vi "Is Control Present.vi"(8 "Error In":errorcluster, 10 "Control label":string, 11 "VI ref":refnum<vi>) -> (0 "Error Out":errorcluster, 2 "Present":bool, 3 "VI ref out":refnum<vi>)   [LabVIEW 2015]
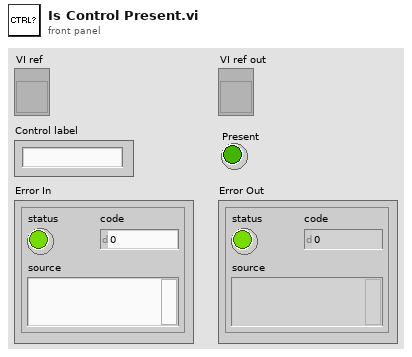
[diagram p1: front panel]
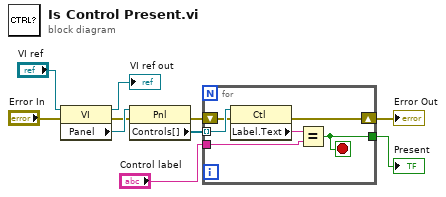
[diagram p0: block diagram]
diagram:
  n1 = property class="VI"(reference="VI ref", error in="Error In") -> (reference out=→"VI ref out":refnum<vi>, error out=w6:errorcluster, "Panel"=w9:refnum<vi>)
  n2 = property class="Pnl"(reference=w9, error in=w6) -> (error out=w5:errorcluster, "Controls[]"=w8:refnum<vi>[])  [unwired: 1 out]
  n3 = for {
    tunnel: w8 -> [w16] mode=indexing
    shift-right: [w14] -> w3
    shift-left: w5 -> [w15]
    tunnel: "Control label" -> [w12]
    tunnel: [w11] -> w2
    stop <- w11 stop-if-true
    n4 = property class="Ctl"(reference=w16, error in=w15) -> (error out=w14:errorcluster, "Label.Text"=w13:string)  [unwired: 1 out]
    n5 = Equal?(x=w13, y=w12) -> (x = y?=w11:bool)
  }
  "Error Out" <- w3
  "Present" <- w2
